vi "SyncTracepoints.vi"(8 "error in (no error)":errorcluster, 11 "new tracepoints":T1[](array[typedef])) -> (0 "error out":errorcluster)   [LabVIEW 2017, in "TraceLogger.lvlib"]
uses:
  <vilib>/addons/TraceLogger/TraceLogger.lvlib
  <vilib>/addons/TraceLogger/controls/TracepointConfig.ctl
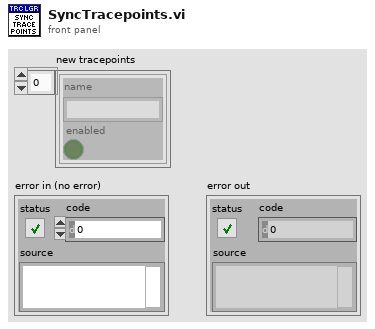
[diagram p1: front panel]
types:
  T1 = typedef "TraceLogger.lvlib/TracepointConfig.ctl" = cluster{"name":string, "enabled":bool}
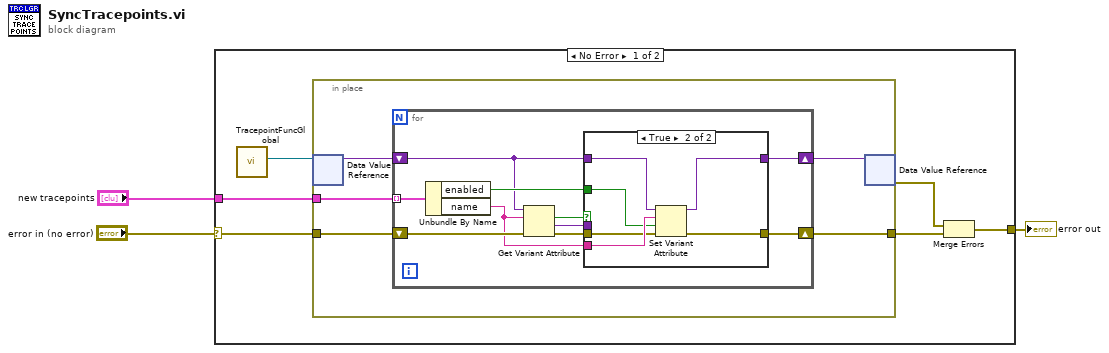
[diagram p0: block diagram]
diagram:
  n1 = case shown="No Error" "error in (no error)" {
    selector: "error in (no error)" -> [w4 w33]
    tunnel: "new tracepoints" -> [w9 _]
    tunnel: [w6 w33] -> w2
    frame No Error {
      n2 = call <vilib>:"TracepointFuncGlobal.vi"() -> ("tracepoints"=w8:refnum<data-value>)  [unwired: 11 in]
      n3 = in-place {
        in-place-border: w4 -> [w14]
        in-place-border: w9 -> [w13]
        in-place-border: [w12] -> w5
        n4 = in-place-dvr #1(w8) -> (w11:variant)  [unwired: 1 out]
        n5 = for {
          tunnel: w13 -> [w23] mode=indexing
          shift-right: [w17] -> w10
          shift-left: w11 -> [w18]
          shift-right: [w15] -> w12
          shift-left: w14 -> [w24]
          n6 = Unbundle By Name(w23) -> ("enabled"=w21:bool, "name"=w16:string)
          n7 = Get Variant Attribute(Variant=w18, name=w16, error in=w24) -> (found=w22:bool, value=w19:variant, error out=w20:errorcluster)  [unwired: 1 in, 1 out]
          n8 = case shown="True" w22 {
            tunnel: w21 -> [_ w27]
            tunnel: w20 -> [w26 w28]
            tunnel: w19 -> [_ _]
            tunnel: w18 -> [w25 w32]
            tunnel: [w25 w31] -> w17
            tunnel: w16 -> [_ w30]
            tunnel: [w26 w29] -> w15
            frame False {
            }
            frame True {
              n9 = Set Variant Attribute(Variant=w32, name=w30, value=w27, error in=w28) -> (Variant out=w31:variant, error out=w29:errorcluster)  [unwired: 1 out]
            }
          }
        }
        n10 = in-place-dvr #1(w10) -> (w7:errorcluster)  [unwired: 1 out]
      }
      n11 = Merge Errors(w7, w5) -> (w6:errorcluster)
    }
    frame Error {
    }
  }
  "error out" <- w2
